vi "updateEditedTimes.vi"(8 "error in (no error)":errorcluster, 11 "ScriptEventList in":refnum<class "ScriptEventList.lvclass">) -> (0 "error out":errorcluster, 3 "ScriptEventList out":refnum<class "ScriptEventList.lvclass">)   [LabVIEW 2011, in "Tools.lvlib" / "Scripting.lvlib" / "ScriptEventList.lvclass"]
uses:
  ScriptEventList.lvclass
  ScriptEventList.lvclass/ScriptEventList.ctl
  ScriptEvent.lvclass
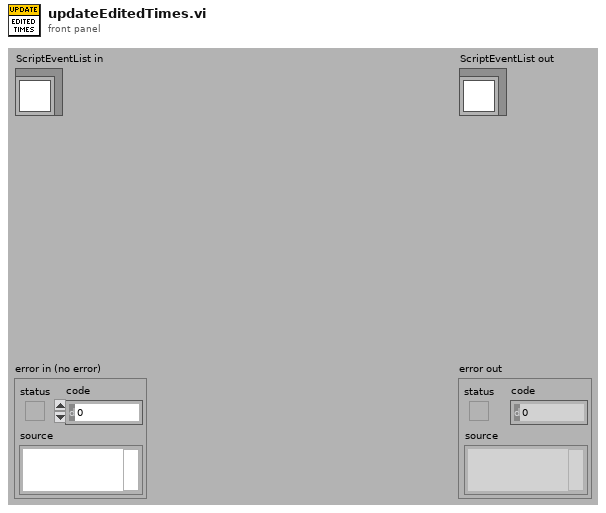
[diagram p1: front panel]
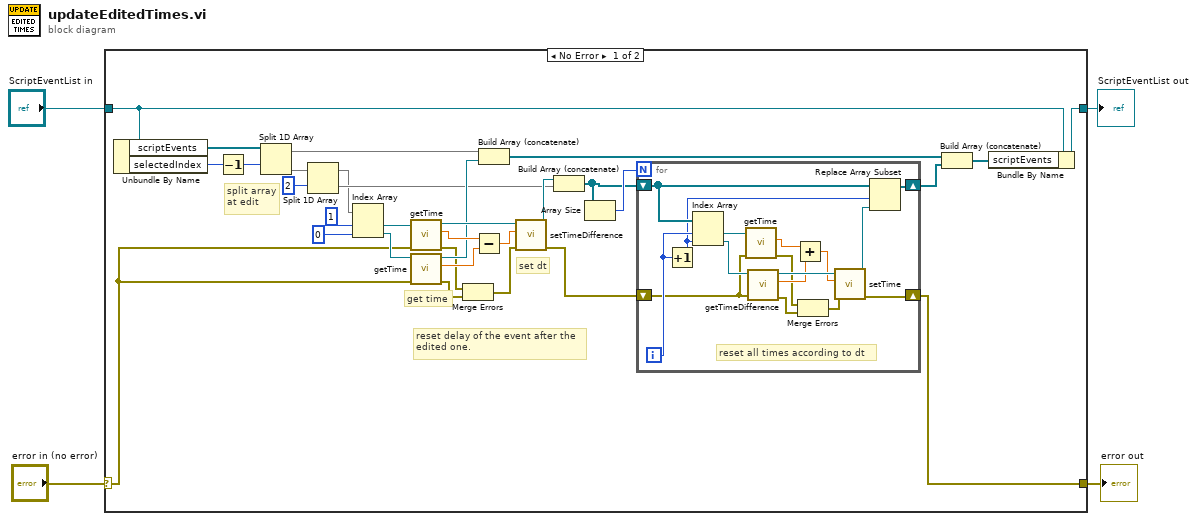
[diagram p0: block diagram]
diagram:
  n1 = case shown="No Error" "error in (no error)" {
    selector: "error in (no error)" -> [w27 w53]
    tunnel: [w6 w53] -> w3
    tunnel: [w7 w52] -> w1
    tunnel: "ScriptEventList in" -> [w8 w52]
    frame No Error {
      # "reset delay of the event after the\nedited one."
      # "split array\nat edit"
      # "set dt"
      # "get time"
      n2 = Unbundle By Name(w8) -> ("scriptEvents"=w33:refnum<class "ScriptEvent.lvclass">[], "selectedIndex"=w35:i32)
      n3 = Decrement(x=w35) -> (x-1=w34:i32)
      n4 = Split 1D Array(array=w33, index=w34) -> (first subarray=w22:refnum<class "ScriptEvent.lvclass">[], second subarray=w32:refnum<class "ScriptEvent.lvclass">[])
      n5 = Split 1D Array(array=w32, index=2) -> (first subarray=w16:refnum<class "ScriptEvent.lvclass">[], second subarray=w17:refnum<class "ScriptEvent.lvclass">[])
      n6 = Index Array(array=w16, index #1=1, index #2=0) -> (element #1=w29:refnum<class "ScriptEvent.lvclass">, element #2=w28:refnum<class "ScriptEvent.lvclass">)
      n7 = call "getTime.vi"("error in (no error)"=w27, "ScriptEvent.lvclass in"=w29) -> ("error out"=w20:errorcluster, "time"=w25:dbl, "ScriptEvent.lvclass out"=w23:refnum<class "ScriptEvent.lvclass">)  [unwired: 7 in]
      n8 = call "getTime.vi"("error in (no error)"=w27, "ScriptEvent.lvclass in"=w28) -> ("error out"=w19:errorcluster, "time"=w26:dbl, "ScriptEvent.lvclass out"=w21:refnum<class "ScriptEvent.lvclass">)  [unwired: 7 in]
      n9 = Merge Errors(w20, w19) -> (w15:errorcluster)
      n10 = Subtract(x=w25, y=w26) -> (x-y=w24:dbl)
      n11 = Build Array (concatenate)(w22, w21) -> (w11:refnum<class "ScriptEvent.lvclass">[])
      n12 = call "setTimeDifference.vi"("error in (no error)"=w15, "time difference"=w24, "ScriptEvent.lvclass in"=w23) -> ("error out"=w12:errorcluster, "ScriptEvent.lvclass out"=w18:refnum<class "ScriptEvent.lvclass">)  [unwired: 7 in]
      n13 = Build Array (concatenate)(w18, w17) -> (w13:refnum<class "ScriptEvent.lvclass">[])
      n14 = Array Size(array=w13) -> (size(s)=w14:i32)
      n15 = for {
        N: w14 -> [_]
        shift-right: [w36] -> w10
        shift-left: w13 -> [w39]
        shift-right: [w40] -> w6
        shift-left: w12 -> [w48]
        i -> [w51]
        # "reset all times according to dt"
        n16 = Increment(x=w51) -> (x+1=w38:i32)
        n17 = Index Array(array=w39, index #1=w51, index #2=w38) -> (element #1=w50:refnum<class "ScriptEvent.lvclass">, element #2=w49:refnum<class "ScriptEvent.lvclass">)
        n18 = call "getTime.vi"("error in (no error)"=w48, "ScriptEvent.lvclass in"=w50) -> ("error out"=w43:errorcluster, "time"=w46:dbl)  [unwired: 7 in, 1 out]
        n19 = call "getTimeDifference.vi"("error in (no error)"=w48, "ScriptEvent.lvclass in"=w49) -> ("error out"=w42:errorcluster, "time difference"=w45:dbl, "ScriptEvent.lvclass out"=w47:refnum<class "ScriptEvent.lvclass">)  [unwired: 7 in]
        n20 = Add(x=w46, y=w45) -> (x+y=w44:dbl)
        n21 = Merge Errors(w43, w42) -> (w41:errorcluster)
        n22 = call "setTime.vi"("error in (no error)"=w41, "time"=w44, "ScriptEvent.lvclass in"=w47) -> ("error out"=w40:errorcluster, "ScriptEvent.lvclass out"=w37:refnum<class "ScriptEvent.lvclass">)  [unwired: 7 in]
        n23 = Replace Array Subset(array=w39, new element=w37, index=w38) -> (w36:refnum<class "ScriptEvent.lvclass">[])
      }
      n24 = Build Array (concatenate)(w11, w10) -> (w9:refnum<class "ScriptEvent.lvclass">[])
      n25 = Bundle By Name(cluster=w8, "scriptEvents"=w9) -> (w7:refnum<class "ScriptEventList.lvclass">)
    }
    frame Error {
    }
  }
  "error out" <- w3
  "ScriptEventList out" <- w1
